vi "SimpleEndpointController.vi"(3 "error in":errorcluster, 4 "Controls":T2={"Rotation"=-42.91139240506329, "Distance"=17.78481012658228, "Wrist"=-20.886075949367083, "Height"=0.25316455696202533, "Hand Orientation"=enum."Down"} {"Height" scale=-10.0..10.0; "Wrist" scale=-90.0..90.0; "Distance" scale=10.0..25.0; "Rotation" scale=-60.0..60.0}, 5 "Side":T1=enum."right") -> (0 "error out":errorcluster)   [LabVIEW 2012]
doc: "A simple endpoint controller for Baxter's hand"
uses:
  <userlib>/rosforlv/ROS/Code/SubVIs/BaxterArmsSmall.ctl
  <userlib>/rosforlv/ROS/Code/SubVIs/BaxterSide.ctl
  <userlib>/rosforlv/ROS/Code/SubVIs/JointMode.ctl
panel:
  out "g":dbl=49.666540029773564
  out "x":dbl=17.786611918279583
  out "p":dbl=0.8155432028971262
  out "a":dbl=54.75975470538772
  in  "Start":T3={"Elbow 0"=0.0, "Elbow 1"=55.8123726628928, "Shoulder 0"=0.0, "Shoulder 1"=-28.952431226064945, "Wrist 0"=0.0, "Wrist 1"=63.14005856317215, "Wrist 2"=0.0}
  out "Arm Angles (degrees)":T3={"Elbow 0"=0.0, "Elbow 1"=104.42629473516128, "Shoulder 0"=-42.91139240506329, "Shoulder 1"=-55.575297908284846, "Wrist 0"=0.0, "Wrist 1"=41.14900317312356, "Wrist 2"=-20.886075949367083}
  in  "d 4":dbl=10.0
  in  "d 3":dbl=15.0
  in  "d 2":dbl=14.0
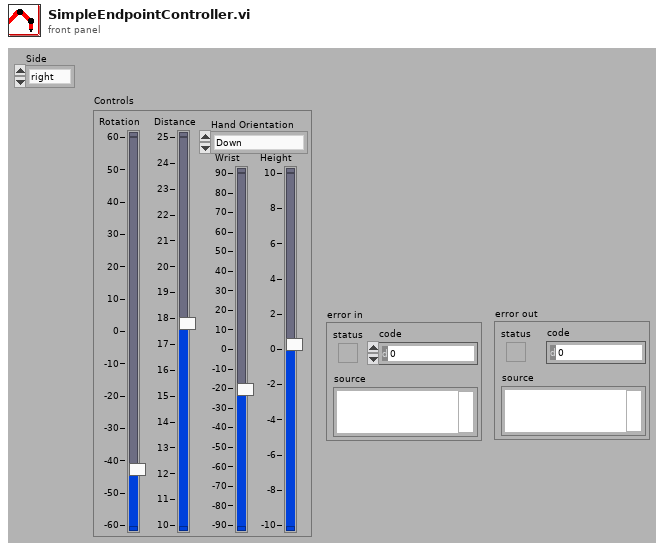
[diagram p1: front panel]
types:
  T1 = typedef "BaxterSide.ctl" = enum16{"left", "right"}
  T2 = cluster{"Rotation":dbl, "Distance":dbl, "Wrist":dbl, "Height":dbl, "Hand Orientation":enum16{"Down", "Flat"}}
  T3 = typedef "BaxterArmsSmall.ctl" = cluster{"Elbow 0":dbl, "Elbow 1":dbl, "Shoulder 0":dbl, "Shoulder 1":dbl, "Wrist 0":dbl, "Wrist 1":dbl, "Wrist 2":dbl}
  T4 = typedef "JointMode.ctl" = u8
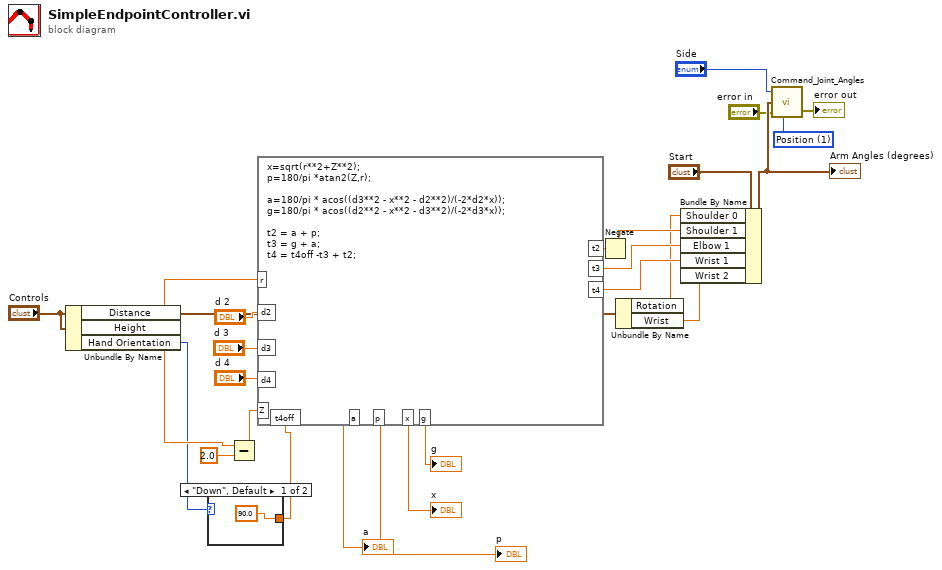
[diagram p0: block diagram]
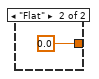
[diagram p2: hidden frame]
diagram:
  w4 = T4 1 items=["Position"=1, "Velocity"=2, "Effort"=3] ("Mode")
  n1 = Unbundle By Name("Controls") -> ("Distance"=w10:dbl, "Height"=w9:dbl, "Hand Orientation"=w8:enum16{"Down", "Flat"})
  n2 = case shown="\"Down\", Default" w8 {
    tunnel: [90.0 ("y") 0.0 ("y")] -> w11
    frame "Down", Default {
    }
    frame "Flat" {
    }
  }
  n3 = Subtract(x=w9, y=2.0) -> (x-y=w12:dbl)
  n4 = formula code="x=sqrt(r**2+Z**2);\np=180/pi *atan2(Z,r);\n\na=180/pi * acos((d3**2 - x**2 - d2**2)/(-2*d2*x));\ng=180/pi * acos((d2**2 - x**2 - d3**2)/(-2*d3*x));\n\nt2 = a + p;\nt3 = g + a;\nt4 = t4off -t3 + t2;"("r"=w10, "d2"="d 2", "d3"="d 3", "d4"="d 4", "Z"=w12, "t4off"=w11) -> ("t2"=w21:dbl, "t3"=w20:dbl, "t4"=w19:dbl, "a"=→"a":dbl, "p"=→"p":dbl, "x"=→"x":dbl, "g"=→"g":dbl)
  n5 = Negate(x=w21) -> (-x=w14:dbl)
  n6 = Unbundle By Name("Controls") -> ("Rotation"=w6:dbl, "Wrist"=w5:dbl)
  n7 = Bundle By Name(cluster="Start", "Shoulder 0"=w6, "Shoulder 1"=w14, "Elbow 1"=w20, "Wrist 1"=w19, "Wrist 2"=w5) -> (w25:T3)
  "Arm Angles (degrees)" <- w25
  n8 = call <userlib>:"Command_Joint_Angles.vi"("Side"="Side", "Arm Angles (degrees)"=w25, "error in"="error in", "Mode"=w4) -> ("error out"=→"error out":errorcluster)  [unwired: 2 in]
